vi "run_weather.vi"() -> ()   [LabVIEW 2011]
uses:
  <vilib>/xml/Load XML File.vi
  <vilib>/xml/Close Reference(Node).vi
  Dependencies/global.vi
  <vilib>/xml/NI_XML.lvlib
panel:
  out "SolarRadiation":string
  out "Error File Write":errorcluster
  out "Error Image Convert":errorcluster
  out "+4 Day Hourly Forecast":string[][](array[string])
  out "+3 Day Hourly Forecast":string[][](array[string])
  out "+2 Day Hourly Forecast":string[][](array[string])
  out "+1 Day Hourly Forecast":string[][](array[string])
  in  "File Path":string="C:\\HVAC\\weather.xml"
  out "Error Msg":string
  out "Updating Weather":bool
  out "?":picture
  out "Today Hourly Forecast":string[][](array[string])
  in  "Update Interval (minutes)":dbl=30.0
  out "Now":string[][](array[string])
  out "Observation Time (RFC 822)":string
  out "Elevation":string
  out "Longitude":string
  out "Latitude":string
  out "Country (ISO 3166)":string
  out "Location":string
  in  "City":string="stockholm"
  in  "Country":string="sweden"
  out "URL":string
  out "Key ID":string="3b63fd7c50251341"
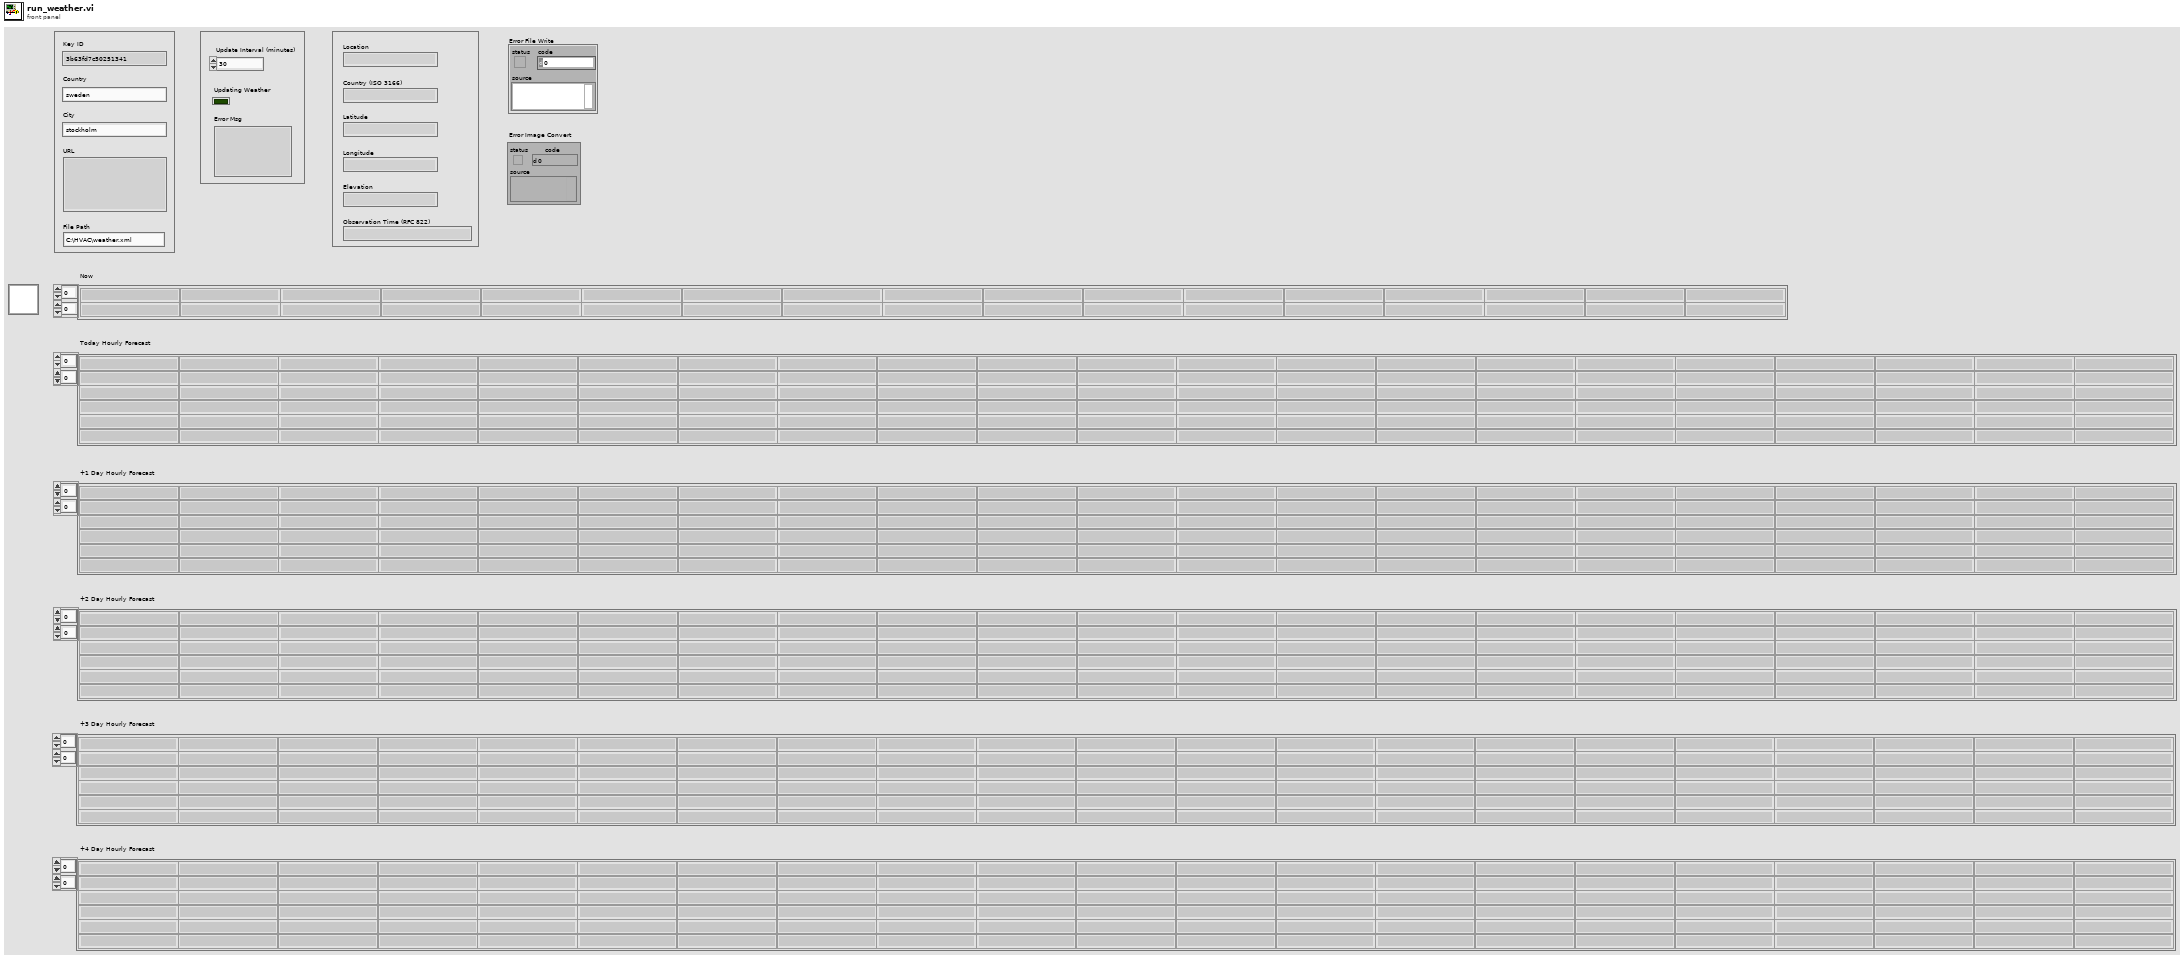
[diagram p1: front panel]
types:
  T1 = cluster{string, string, string, string, string, string, string, string}
  T2 = enum16{"open", "open or create", "create or replace", "create", "open (read only)"}
  T3 = typedef "imagedata.ctl" = cluster{"image type":i32, "image depth":i32, "image":u8[], "mask":u8[], "colors":u32[], "Rectangle":cluster{"left":i16, "top":i16, "right":i16, "bottom":i16}}
  T4 = cluster{string, string, string, string, string, "date/time string":string, string, string}
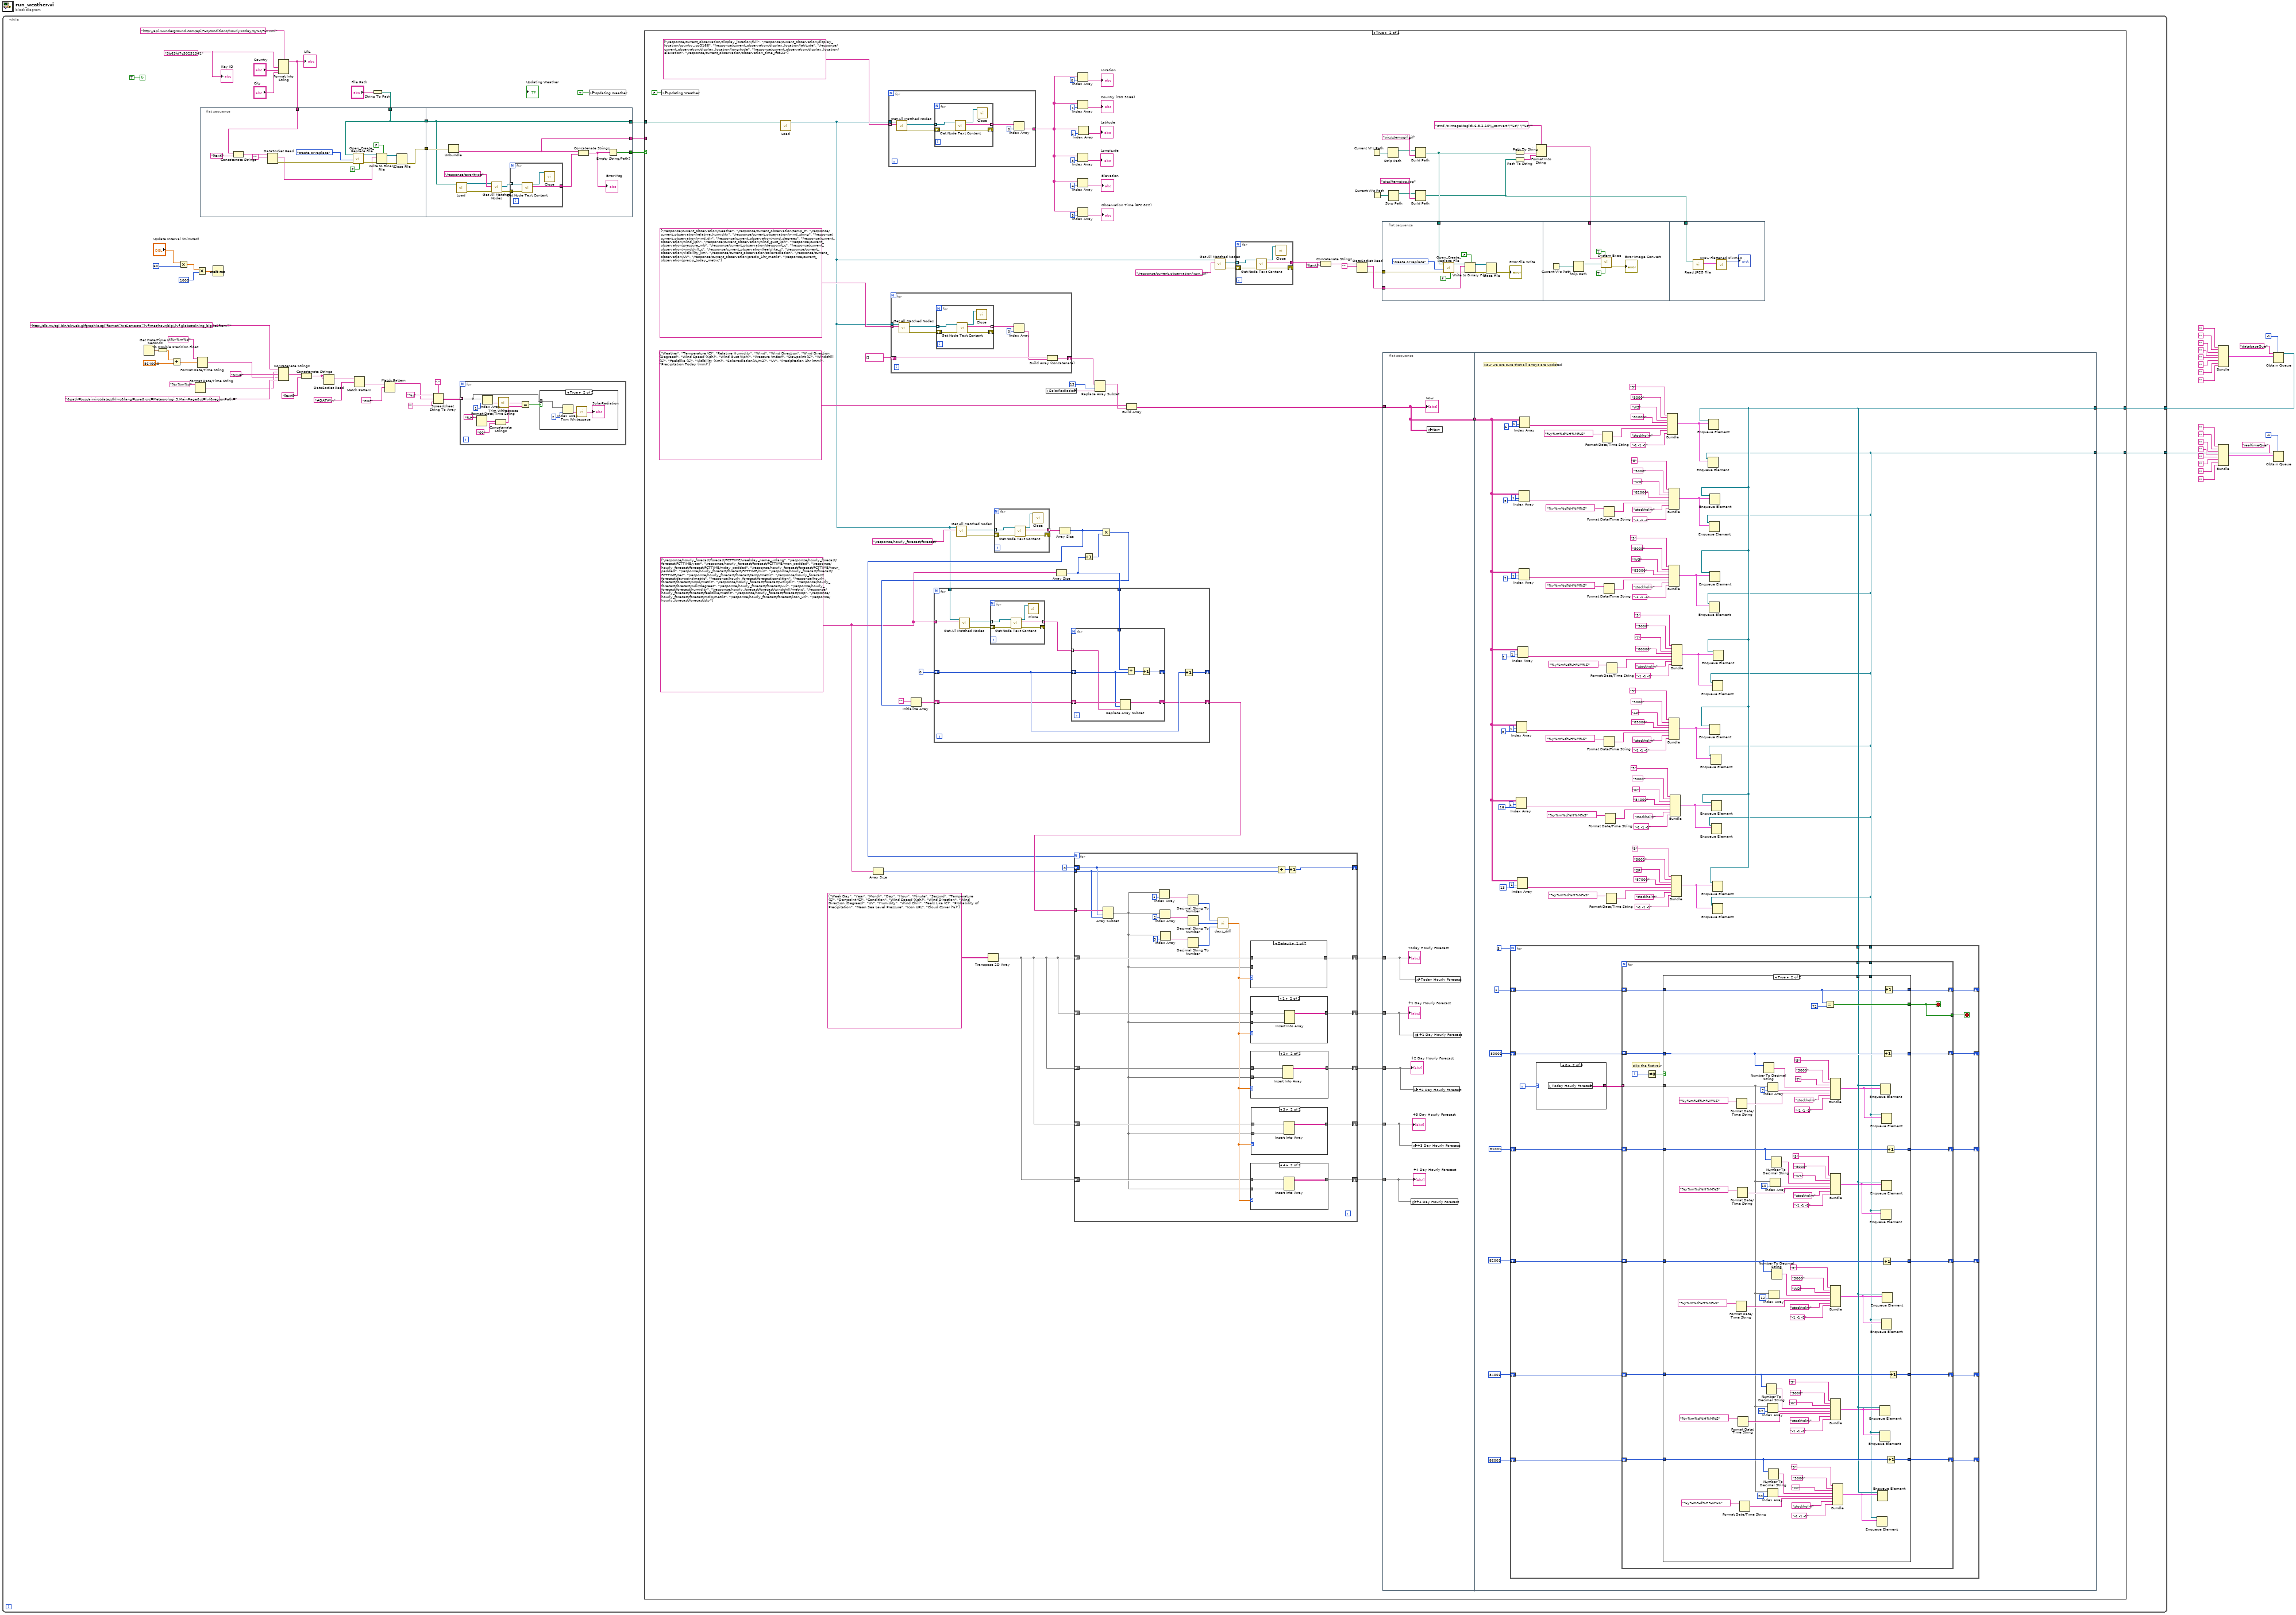
[diagram p0: block diagram]
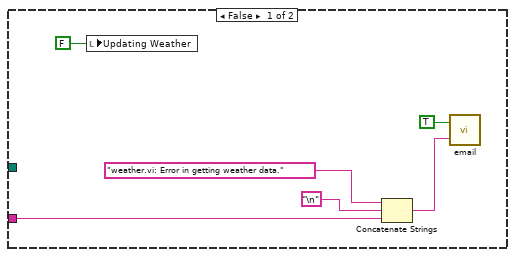
[diagram p3: hidden frame]
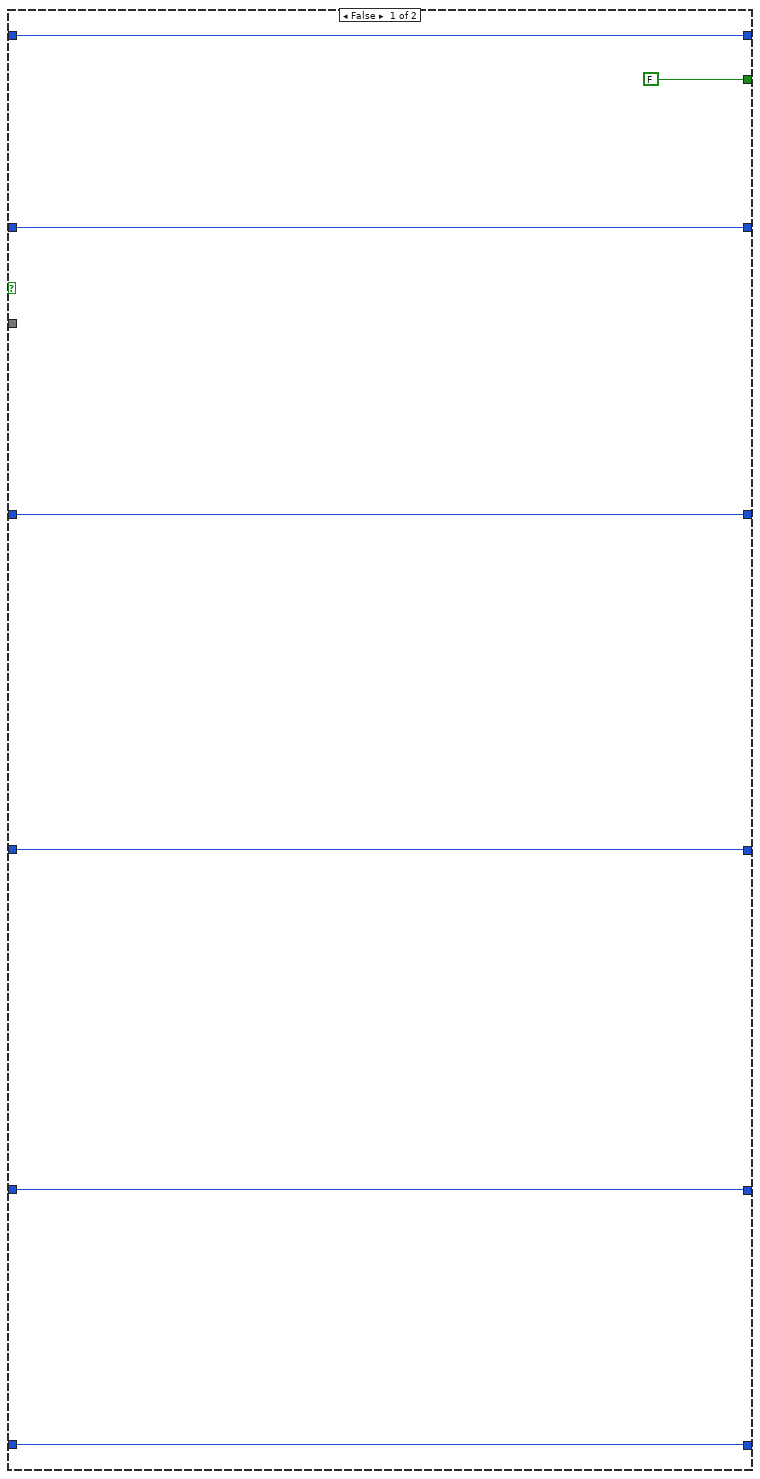
[diagram p4: hidden frame]
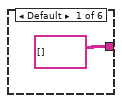
[diagram p5: hidden frame]
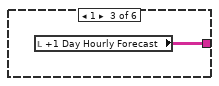
[diagram p6: hidden frame]
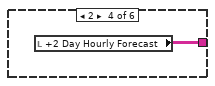
[diagram p7: hidden frame]
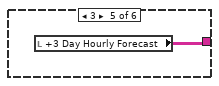
[diagram p8: hidden frame]
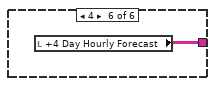
[diagram p9: hidden frame]
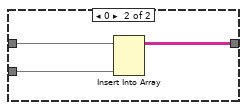
[diagram p14: hidden frame]
diagram:
  n1 = Bundle("", "", "", "", "", "", "", "") -> (w17:T1)  [unwired: 1 in]
  n2 = Bundle("", "", "", "", "", "", "", "") -> (w6:T1)  [unwired: 1 in]
  n3 = Obtain Queue(max queue size (-1, unlimited)=-1, name (unnamed)="databaseQue", element data type=w17) -> (queue out=w2:refnum<queue>)  [unwired: 2 in, 2 out]
  n4 = Obtain Queue(max queue size (-1, unlimited)=-1, name (unnamed)="realtimeQue", element data type=w6) -> (queue out=w1:refnum<queue>)  [unwired: 2 in, 2 out]
  n5 = while {
    tunnel: w2 -> [w49]
    tunnel: w1 -> [w48]
    stop <- TRUE continue-if-true
    w67 = "3b63fd7c50251341"
    n6 = Get Date/Time In Seconds() -> (seconds since 1Jan1904=w34:timestamp)
    n7 = To Double Precision Float(number=w34) -> (double precision float=w33:dbl)
    n8 = Add(x=w33, y=86400.0) -> (x+y=w31:dbl)
    n9 = Multiply(x="Update Interval (minutes)", y=60) -> (x*y=w64:dbl)
    n10 = Format Date/Time String(time format string (%c)="%y%m%d") -> (date/time string=w28:string)  [unwired: 2 in]
    n11 = Multiply(x=w64, y=1000) -> (x*y=w62:dbl)
    n12 = Format Date/Time String(time format string (%c)="%y%m%d", seconds (now)=w31) -> (date/time string=w27:string)  [unwired: 1 in]
    n13 = flat-sequence {
      tunnel: w50 -> [w83]
      tunnel: [w83] -> w57
      tunnel: [w82] -> w56
      tunnel: w53 -> [w86]
      tunnel: w57 -> [w99]
      tunnel: w56 -> [w100]
      tunnel: [w99] -> w55
      tunnel: [w98] -> w54
      tunnel: [w97] -> w52
      frame #0 {
        n14 = Concatenate Strings(w86, "[text]" ("string")) -> (w89:string)
        n15 = DataSocket Read(10:"", 11:w89) -> (0:w85:errorcluster, 2:w84:string)  [unwired: 3 in, 5 out]
        n16 = call <vilib>:"Open_Create_Replace File.vi"("advisory dialog? (display:T)"=FALSE, "error in (no error)"=w85, "function (open:0)"=T2."create or replace", "file path"=w83) -> ("error out"=w92:errorcluster, "refnum"=w91:refnum<file>)  [unwired: 3 in, 3 out]
        n17 = Write to Binary File(file (use dialog)=w91, data=w84, error in=w92, 5:FALSE ("prepend array or string size? (T)")) -> (refnum out=w95:refnum<file>, error out=w96:errorcluster)  [unwired: 3 out]
        n18 = Close File(refnum=w95, error in=w96) -> (error out=w82:errorcluster)  [unwired: 1 out]
      }
      frame #1 {
        n19 = Unbundle(w100) -> ("source"=w97:string)  [unwired: 2 out]
        n20 = call-poly <vilib>:"Load.vi"("path to XML document"=w99) -> ("DOM document out"=w105:refnum<k20>, "error out"=w104:errorcluster)  [unwired: 12 in, 1 out]
        n21 = call <vilib>:"Get All Matched Nodes.vi"("error in (no error)"=w104, "XPath expression"="/response/error/type", "node in"=w105) -> ("error out"=w107:errorcluster, "node result array"=w103:refnum<k20>[])  [unwired: 7 out]
        n22 = for {
          tunnel: w107 -> [w111]
          tunnel: [w110] -> w101
          tunnel: w103 -> [w108] mode=indexing
          n23 = call <vilib>:"Get Node Text Content.vi"("error in (no error)"=w111, "node in"=w108) -> ("node text"=w110:string, "node out"=w109:refnum<k20>)  [unwired: 7 in, 1 out]
          n24 = call-poly <vilib>:"Close.vi"("node"=w109) -> ()  [unwired: 8 in, 1 out]
        }
        n25 = Concatenate Strings(w97, w101) -> (w102:string)
        "Error Msg" <- w102
        n26 = Empty String/Path?(string/path=w102) -> (empty?=w98:bool)
      }
    }
    n27 = Wait (ms)(milliseconds to wait=w62) -> ()  [unwired: 1 out]
    n28 = Format Into String(format string="http://api.wunderground.com/api/%s/conditions/hourly10day/q/%s/%s.xml", w67, "Country", "City") -> (resulting string=w53:string)  [unwired: 2 in, 1 out]
    "URL" <- w53
    n29 = Concatenate Strings("http://slb.nu/cgi-bin/airweb.gifgraphic.cgi?format=txt&zmacro=lvf/met/hour/big//lvf-globstralning_big.ic&from=" ("string"), w28, "&to=" ("string"), w27, "&path=/usr/airviro/data/sthlm/&lang=swe&rsrc=Meteorologi.3.MainPage&st=lvf&regionPath=" ("string")) -> (w38:string)
    n30 = Concatenate Strings(w38, "[text]" ("string")) -> (w46:string)
    n31 = DataSocket Read(10:w46, 11:w46) -> (2:w45:string)  [unwired: 3 in, 6 out]
    n32 = Match Pattern(string=w45, regular expression="#DATA\\n") -> (after substring=w37:string)  [unwired: 1 in, 3 out]
    n33 = String To Path(string="File Path") -> (path=w50:path)
    n34 = Match Pattern(string=w37, regular expression="EOF") -> (before substring=w25:string)  [unwired: 1 in, 3 out]
    n35 = Spreadsheet String To Array(delimiter (Tab)=",", format string="%s", spreadsheet string=w25, array type (2D Dbl)="") -> (array=w26:string[][])
    n36 = for {
      tunnel: w26 -> [w71] mode=indexing
      n37 = Format Date/Time String(time format string (%c)="%H") -> (date/time string=w75:string)  [unwired: 2 in]
      n38 = Index Array(array=w71, index=1) -> (element=w70:string)
      n39 = Concatenate Strings(w75, "00" ("string")) -> (w73:string)
      n40 = call <vilib>:"Trim Whitespace.vi"("string"=w70) -> ("trimmed string"=w69:string)  [unwired: 1 in]
      n41 = Equal?(x=w69, y=w73) -> (x = y?=w72:bool)
      n42 = case shown="True" w72 {
        tunnel: w71 -> [_ w81]
        frame False {
        }
        frame True {
          n43 = Index Array(array=w81, index=2) -> (element=w78:string)
          n44 = call <vilib>:"Trim Whitespace.vi"("string"=w78) -> ("trimmed string"=→"SolarRadiation":string)  [unwired: 1 in]
        }
      }
    }
    n45 = local write "Updating Weather"(TRUE ("Backup in Progress")) -> ()
    n46 = case shown="True" w54 {
      tunnel: w55 -> [_ w188]
      tunnel: w52 -> [w113 _]
      tunnel: w49 -> [_ w123]
      tunnel: w48 -> [_ w122]
      frame False {
        n47 = local write "Updating Weather"(FALSE ("Updating Weather")) -> ()
        n48 = Concatenate Strings("weather.vi: Error in getting weather data.", "\n", w113) -> (w112:string)
        n49 = call "email.vi"("Body"=w112, "Enable"=TRUE) -> ()  [unwired: 1 in]
      }
      frame True {
        w141 = string[] ["/response/hourly_forecast/forecast/FCTTIME/weekday_name_unlang", "/response/hourly_forecast/forecast/FCTTIME/year", "/response/hourly_forecast/forecast/FCTTIME/mon_padded", "/response/hourly_forecast/forecast/FCTTIME/mday_padded", "/response/hourly_forecast/forecast/FCTTIME/hour_padded", "/response/hourly_forecast/forecast/FCTTIME/min", "/response/hourly_forecast/forecast/FCTTIME/sec", "/response/hourly_forecast/forecast/temp/metric", "/response/hourly_forecast/forecast/dewpoint/metric", "/response/hourly_forecast/forecast/condition", "/response/hourly_forecast/forecast/wspd/metric", "/response/hourly_forecast/forecast/wdir/dir", "/response/hourly_forecast/forecast/wdir/degrees", "/response/hourly_forecast/forecast/uvi", "/response/hourly_forecast/forecast/humidity", "/response/hourly_forecast/forecast/windchill/metric", "/response/hourly_forecast/forecast/feelslike/metric", "/response/hourly_forecast/forecast/pop", "/response/hourly_forecast/forecast/mslp/metric", "/response/hourly_forecast/forecast/icon_url", "/response/hourly_forecast/forecast/sky"]
        n50 = local write "Updating Weather"(FALSE ("Backup in Progress")) -> ()
        n51 = call-poly <vilib>:"Load.vi"("path to XML document"=w188) -> ("DOM document out"=w125:refnum<k20>)  [unwired: 12 in, 2 out]
        n52 = Array Size(array=w141) -> (size(s)=w140:i32)
        n53 = for {
          tunnel: string[] ["/response/current_observation/display_location/full", "/response/current_observation/display_location/country_iso3166", "/response/current_observation/display_location/latitude", "/response/current_observation/display_location/longitude", "/response/current_observation/display_location/elevation", "/response/current_observation/observation_time_rfc822"] -> [w526] mode=indexing
          tunnel: w125 -> [w525]
          tunnel: [w521] -> w179 mode=indexing
          n54 = call <vilib>:"Get All Matched Nodes.vi"("XPath expression"=w526, "node in"=w525) -> ("error out"=w524:errorcluster, "node result array"=w527:refnum<k20>[])  [unwired: 1 in, 7 out]
          n55 = for {
            tunnel: w527 -> [w532] mode=indexing
            tunnel: [w531] -> w523 mode=indexing
            shift-right: [w529] -> _
            shift-left: w524 -> [w530]
            n56 = call <vilib>:"Get Node Text Content.vi"("error in (no error)"=w530, "node in"=w532) -> ("error out"=w529:errorcluster, "node text"=w531:string, "node out"=w528:refnum<k20>)  [unwired: 7 in]
            n57 = call-poly <vilib>:"Close.vi"("node"=w528) -> ()  [unwired: 8 in, 1 out]
          }
          n58 = Index Array(array=w523, index=0) -> (element=w521:string)
        }
        n59 = for {
          tunnel: string[] ["/response/current_observation/weather", "/response/current_observation/temp_c", "/response/current_observation/relative_humidity", "/response/current_observation/wind_string", "/response/current_observation/wind_dir", "/response/current_observation/wind_degrees", "/response/current_observation/wind_kph", "/response/current_observation/wind_gust_kph", "/response/current_observation/pressure_mb", "/response/current_observation/dewpoint_c", "/response/current_observation/windchill_c", "/response/current_observation/feelslike_c", "/response/current_observation/visibility_km", "/response/current_observation/solarradiation", "/response/current_observation/UV", "/response/current_observation/precip_1hr_metric", "/response/current_observation/precip_today_metric"] -> [w514] mode=indexing
          shift-right: [w510] -> w121
          shift-left: string[] [] -> [w509]
          tunnel: w125 -> [w507]
          n60 = call <vilib>:"Get All Matched Nodes.vi"("XPath expression"=w514, "node in"=w507) -> ("error out"=w513:errorcluster, "node result array"=w515:refnum<k20>[])  [unwired: 1 in, 7 out]
          n61 = for {
            tunnel: w515 -> [w520] mode=indexing
            tunnel: [w519] -> w512 mode=indexing
            shift-right: [w517] -> _
            shift-left: w513 -> [w518]
            n62 = call <vilib>:"Get Node Text Content.vi"("error in (no error)"=w518, "node in"=w520) -> ("error out"=w517:errorcluster, "node text"=w519:string, "node out"=w516:refnum<k20>)  [unwired: 7 in]
            n63 = call-poly <vilib>:"Close.vi"("node"=w516) -> ()  [unwired: 8 in, 1 out]
          }
          n64 = Index Array(array=w512, index=0) -> (element=w508:string)
          n65 = Build Array (concatenate)(w509, w508) -> (w510:string[])
        }
        n66 = call <vilib>:"Get All Matched Nodes.vi"("XPath expression"="/response/hourly_forecast/forecast", "node in"=w125) -> ("error out"=w168:errorcluster, "node result array"=w167:refnum<k20>[])  [unwired: 1 in, 7 out]
        n67 = Transpose 2D Array(2D array=string[][] [["Week Day"], ["Year"], ["Month"], ["Day"], ["Hour"], ["Minute"], ["Second"], ["Temperature (C)"], ["Dewpoint (C)"], ["Condition"], ["Wind Speed (Kph)"], ["Wind Direction"], ["Wind Direction (Degrees)"], ["UV"], ["Humidity"], ["Wind Chill"], ["Feels Like (C)"], ["Probability of Precipitation"], ["Mean Sea Level Pressure"], ["Icon URL"], ["Cloud Cover (%)"]]) -> (transposed array=w132:string[][])
        n68 = for {
          tunnel: w167 -> [w484] mode=indexing
          tunnel: [w483] -> w165 mode=indexing
          shift-right: [w481] -> _
          shift-left: w168 -> [w482]
          n69 = call <vilib>:"Get Node Text Content.vi"("error in (no error)"=w482, "node in"=w484) -> ("error out"=w481:errorcluster, "node text"=w483:string, "node out"=w480:refnum<k20>)  [unwired: 7 in]
          n70 = call-poly <vilib>:"Close.vi"("node"=w480) -> ()  [unwired: 8 in, 1 out]
        }
        n71 = local read "SolarRadiation"() -> (w120:string)
        n72 = Array Size(array=w141) -> (size(s)=w164:i32)
        n73 = Array Size(array=w165) -> (size(s)=w139:i32)
        n74 = Index Array(array=w179, index=0) -> (element=→"Location":string)
        n75 = Index Array(array=w179, index=1) -> (element=→"Country (ISO 3166)":string)
        n76 = Index Array(array=w179, index=3) -> (element=→"Longitude":string)
        n77 = Index Array(array=w179, index=4) -> (element=→"Elevation":string)
        n78 = Index Array(array=w179, index=5) -> (element=→"Observation Time (RFC 822)":string)
        n79 = Index Array(array=w179, index=2) -> (element=→"Latitude":string)
        n80 = Increment(x=w164) -> (x+1=w163:i32)
        n81 = Replace Array Subset(array=w121, new element=w120, index=13) -> (w118:string[])
        n82 = Multiply(x=w139, y=w163) -> (x*y=w162:i32)
        n83 = Initialize Array("", w162) -> (w169:string[])
        n84 = for {
          tunnel: w141 -> [w493] mode=indexing
          tunnel: w125 -> [w491]
          shift-right: [w485] -> w143
          shift-left: w169 -> [w486]
          tunnel: w164 -> [w489]
          shift-right: [w488] -> _
          shift-left: 0 -> [w487]
          n85 = call <vilib>:"Get All Matched Nodes.vi"("XPath expression"=w493, "node in"=w491) -> ("error out"=w492:errorcluster, "node result array"=w494:refnum<k20>[])  [unwired: 1 in, 7 out]
          n86 = for {
            tunnel: w494 -> [w506] mode=indexing
            tunnel: [w505] -> w490 mode=indexing
            shift-right: [w503] -> _
            shift-left: w492 -> [w504]
            n87 = call <vilib>:"Get Node Text Content.vi"("error in (no error)"=w504, "node in"=w506) -> ("error out"=w503:errorcluster, "node text"=w505:string, "node out"=w502:refnum<k20>)  [unwired: 7 in]
            n88 = call-poly <vilib>:"Close.vi"("node"=w502) -> ()  [unwired: 8 in, 1 out]
          }
          n89 = for {
            tunnel: w490 -> [w495] mode=indexing
            shift-right: [w499] -> _
            shift-left: w487 -> [w497]
            tunnel: w489 -> [w501]
            shift-right: [w496] -> w485
            shift-left: w486 -> [w498]
            n90 = Replace Array Subset(array=w498, new element=w495, index=w497) -> (w496:string[])
            n91 = Add(x=w501, y=w497) -> (x+y=w500:i32)
            n92 = Increment(x=w500) -> (x+1=w499:i32)
          }
          n93 = Increment(x=w487) -> (x+1=w488:i32)
        }
        n94 = for {
          N: w139 -> [_]
          tunnel: w143 -> [w434]
          shift-right: [w423] -> w137
          shift-left: w132 -> [w424]
          shift-right: [w421] -> w138
          shift-left: w132 -> [w422]
          shift-right: [w419] -> _
          shift-left: u64 0 -> [w418]
          tunnel: w140 -> [w417]
          shift-right: [w412] -> w136
          shift-left: w132 -> [w415]
          shift-right: [w411] -> w135
          shift-left: w132 -> [w414]
          shift-right: [w410] -> w134
          shift-left: w132 -> [w413]
          n95 = Array Subset(array=w434, index=w418, length=w417) -> (w409:string[])
          n96 = Index Array(array=w409, index=1 ("index (row)")) -> (element=w430:string)
          n97 = Index Array(array=w409, index=2 ("index (row)")) -> (element=w429:string)
          n98 = Index Array(array=w409, index=3 ("index (row)")) -> (element=w428:string)
          n99 = Decimal String To Number(string=w430) -> (number=w427:i32)  [unwired: 2 in, 1 out]
          n100 = Decimal String To Number(string=w429) -> (number=w426:i32)  [unwired: 2 in, 1 out]
          n101 = Decimal String To Number(string=w428) -> (number=w425:i32)  [unwired: 2 in, 1 out]
          n102 = call "days_diff.vi"("day"=w425, "month"=w426, "year"=w427) -> ("Days Diff"=w416:dbl)  [unwired: 2 out]
          n103 = case shown="Default" w416 {
            tunnel: w424 -> [w451 w454]
            tunnel: w409 -> [_ w453]
            tunnel: [w451 w452] -> w423
            frame Default {
            }
            frame 0 {
              n104 = Insert Into Array(array=w454, new element=w453) -> (w452:string[][])  [unwired: 2 in]
            }
          }
          n105 = case shown="1" w416 {
            tunnel: w422 -> [w447 w450]
            tunnel: w409 -> [_ w449]
            tunnel: [w447 w448] -> w421
            frame Default {
            }
            frame 1 {
              n106 = Insert Into Array(array=w450, new element=w449) -> (w448:string[][])  [unwired: 2 in]
            }
          }
          n107 = case shown="4" w416 {
            tunnel: w413 -> [w435 w438]
            tunnel: w409 -> [_ w437]
            tunnel: [w435 w436] -> w410
            frame Default {
            }
            frame 4 {
              n108 = Insert Into Array(array=w438, new element=w437) -> (w436:string[][])  [unwired: 2 in]
            }
          }
          n109 = case shown="2" w416 {
            tunnel: w415 -> [w443 w446]
            tunnel: w409 -> [_ w445]
            tunnel: [w443 w444] -> w412
            frame Default {
            }
            frame 2 {
              n110 = Insert Into Array(array=w446, new element=w445) -> (w444:string[][])  [unwired: 2 in]
            }
          }
          n111 = case shown="3" w416 {
            tunnel: w414 -> [w439 w442]
            tunnel: w409 -> [_ w441]
            tunnel: [w439 w440] -> w411
            frame Default {
            }
            frame 3 {
              n112 = Insert Into Array(array=w442, new element=w441) -> (w440:string[][])  [unwired: 2 in]
            }
          }
          n113 = Add(x=w418, y=w417) -> (x+y=w420:u64)
          n114 = Increment(x=w420) -> (x+1=w419:u64)
        }
        n115 = Build Array(string[] ["Weather", "Temperature (C)", "Relative Humidity", "Wind", "Wind Direction", "Wind Direction (Degrees)", "Wind Speed (Kph)", "Wind Gust (Kph)", "Pressure (mBar)", "Dewpoint (C)", "Windchill (C)", "Feelslike (C)", "Visibility (Km)", "Solarradiation(W/m2)", "UV", "Precipitation 1hr (mm)", "Precipitation Today (mm)"], w118) -> (w126:string[][])
        n116 = call <vilib>:"Get All Matched Nodes.vi"("XPath expression"="/response/current_observation/icon_url", "node in"=w125) -> ("error out"=w161:errorcluster, "node result array"=w160:refnum<k20>[])  [unwired: 1 in, 7 out]
        n117 = for {
          tunnel: w160 -> [w479] mode=indexing
          tunnel: [w478] -> w155
          shift-right: [w476] -> _
          shift-left: w161 -> [w477]
          n118 = call <vilib>:"Get Node Text Content.vi"("error in (no error)"=w477, "node in"=w479) -> ("error out"=w476:errorcluster, "node text"=w478:string, "node out"=w475:refnum<k20>)  [unwired: 7 in]
          n119 = call-poly <vilib>:"Close.vi"("node"=w475) -> ()  [unwired: 8 in, 1 out]
        }
        n120 = Concatenate Strings(w155, "[text]" ("string")) -> (w153:string)
        n121 = DataSocket Read(10:"", 11:w153) -> (0:w156:errorcluster, 2:w158:string)  [unwired: 3 in, 5 out]
        n122 = Current VI's Path() -> (path=w131:path)
        n123 = Current VI's Path() -> (path=w129:path)
        n124 = flat-sequence {
          tunnel: w158 -> [w463]
          tunnel: w156 -> [w460]
          tunnel: w150 -> [w456]
          tunnel: w145 -> [w467]
          tunnel: w147 -> [w472]
          frame #0 {
            n125 = call <vilib>:"Open_Create_Replace File.vi"("advisory dialog? (display:T)"=FALSE, "error in (no error)"=w460, "function (open:0)"=T2."create or replace", "file path"=w456) -> ("error out"=w462:errorcluster, "refnum"=w464:refnum<file>)  [unwired: 3 in, 3 out]
            n126 = Write to Binary File(file (use dialog)=w464, data=w463, error in=w462, 5:FALSE ("prepend array or string size? (T)")) -> (refnum out=w458:refnum<file>, error out=w457:errorcluster)  [unwired: 3 out]
            n127 = Close File(refnum=w458, error in=w457) -> (error out=→"Error File Write":errorcluster)  [unwired: 1 out]
          }
          frame #1 {
            n128 = Current VI's Path() -> (path=w468:path)
            n129 = Strip Path(path=w468) -> (stripped path=w471:path)  [unwired: 1 out]
            n130 = call <vilib>:"System Exec.vi"("run minimized? (F)"=TRUE, "wait until completion? (T)"=TRUE, "working directory"=w471, "command line"=w467) -> ("error out"=→"Error Image Convert":errorcluster)  [unwired: 4 in, 3 out]
          }
          frame #2 {
            n131 = call <vilib>:"Read JPEG File.vi"("path to JPEG file"=w472) -> ("image data"=w473:T3)  [unwired: 8 in, 2 out]
            n132 = call <vilib>:"Draw Flattened Pixmap.vi"("image data"=w473) -> ("new picture"=→"?":picture)  [unwired: 3 in, 5 out]
          }
        }
        n133 = flat-sequence {
          tunnel: w138 -> [w194]
          tunnel: w137 -> [w193]
          tunnel: w136 -> [w192]
          tunnel: w135 -> [w191]
          tunnel: w134 -> [w190]
          tunnel: w126 -> [w189]
          tunnel: [w189] -> w124
          tunnel: w124 -> [w197]
          tunnel: w123 -> [w196]
          tunnel: w122 -> [w195]
          frame #0 {
            n134 = global write "global.vi" "+4 Day Hourly Forecast"(w190) -> ()
            n135 = global write "global.vi" "+3 Day Hourly Forecast"(w191) -> ()
            n136 = global write "global.vi" "+2 Day Hourly Forecast"(w192) -> ()
            n137 = global write "global.vi" "+1 Day Hourly Forecast"(w194) -> ()
            n138 = global write "global.vi" "Today Hourly Forecast"(w193) -> ()
            n139 = global write "global.vi" "Now"(w189) -> ()
            "Now" <- w189
            "Today Hourly Forecast" <- w193
            "+1 Day Hourly Forecast" <- w194
            "+2 Day Hourly Forecast" <- w192
            "+3 Day Hourly Forecast" <- w191
            "+4 Day Hourly Forecast" <- w190
          }
          frame #1 {
            # "Now we are sure that all arrays are updated"
            n140 = for {
              N: 5 -> [_]
              shift-right: [w301] -> _
              shift-left: 80001 -> [w302]
              tunnel: w196 -> [w304]
              shift-right: [w299] -> _
              shift-left: 81001 -> [w300]
              shift-right: [w297] -> _
              shift-left: 82001 -> [w298]
              shift-right: [w295] -> _
              shift-left: 84001 -> [w296]
              shift-right: [w293] -> _
              shift-left: 1 -> [w294]
              shift-right: [w291] -> _
              shift-left: 86001 -> [w290]
              tunnel: w195 -> [w289]
              i -> [w305]
              stop <- w292 stop-if-true
              n141 = case shown="0" w305 {
                tunnel: [string[][] [] ("Today Hourly Forecast") w404 w405 w406 w407 w408] -> w303
                frame Default {
                }
                frame 0 {
                  n142 = local read "Today Hourly Forecast"() -> (w404:string[][])
                }
                frame 1 {
                  n143 = local read "+1 Day Hourly Forecast"() -> (w405:string[][])
                }
                frame 2 {
                  n144 = local read "+2 Day Hourly Forecast"() -> (w406:string[][])
                }
                frame 3 {
                  n145 = local read "+3 Day Hourly Forecast"() -> (w407:string[][])
                }
                frame 4 {
                  n146 = local read "+4 Day Hourly Forecast"() -> (w408:string[][])
                }
              }
              n147 = for {
                tunnel: w304 -> [w321]
                tunnel: w303 -> [w320] mode=indexing
                shift-right: [w318] -> w301
                shift-left: w302 -> [w319]
                shift-right: [w316] -> w299
                shift-left: w300 -> [w317]
                shift-right: [w315] -> w297
                shift-left: w298 -> [w314]
                shift-right: [w313] -> w295
                shift-left: w296 -> [w312]
                shift-right: [w310] -> w293
                shift-left: w294 -> [w311]
                tunnel: [w309] -> w292
                shift-right: [w307] -> w291
                shift-left: w290 -> [w308]
                tunnel: w289 -> [w306]
                i -> [w323]
                stop <- w309 stop-if-true
                # "skip the first row"
                n148 = Not Equal To 0?(x=w323) -> (x != 0?=w322:bool)
                n149 = case shown="True" w322 {
                  tunnel: [w330 w401] -> w318
                  tunnel: w319 -> [w330 w397]
                  tunnel: w321 -> [_ w338]
                  tunnel: w320 -> [_ w337]
                  tunnel: w317 -> [w329 w392]
                  tunnel: [w329 w391] -> w316
                  tunnel: [w328 w386] -> w315
                  tunnel: w314 -> [w328 w385]
                  tunnel: [w327 w380] -> w313
                  tunnel: w312 -> [w327 w379]
                  tunnel: w311 -> [w326 w376]
                  tunnel: [w326 w377] -> w310
                  tunnel: [FALSE w375] -> w309
                  tunnel: w308 -> [w324 w340]
                  tunnel: [w324 w339] -> w307
                  tunnel: w306 -> [_ w331]
                  frame False {
                  }
                  frame True {
                    n150 = Format Date/Time String(time format string (%c)="%y%m%d%H%M%S") -> (date/time string=w368:string)  [unwired: 2 in]
                    n151 = Format Date/Time String(time format string (%c)="%y%m%d%H%M%S") -> (date/time string=w373:string)  [unwired: 2 in]
                    n152 = Format Date/Time String(time format string (%c)="%y%m%d%H%M%S") -> (date/time string=w369:string)  [unwired: 2 in]
                    n153 = Format Date/Time String(time format string (%c)="%y%m%d%H%M%S") -> (date/time string=w367:string)  [unwired: 2 in]
                    n154 = Format Date/Time String(time format string (%c)="%y%m%d%H%M%S") -> (date/time string=w345:string)  [unwired: 2 in]
                    n155 = Number To Decimal String(number=w397) -> (decimal integer string=w363:string)  [unwired: 1 in]
                    n156 = Number To Decimal String(number=w379) -> (decimal integer string=w351:string)  [unwired: 1 in]
                    n157 = Index Array(array=w337, index=17) -> (element=w384:string)
                    n158 = Index Array(array=w337, index=20) -> (element=w350:string)
                    n159 = Index Array(array=w337, index=7) -> (element=w398:string)
                    n160 = Number To Decimal String(number=w340) -> (decimal integer string=w341:string)  [unwired: 1 in]
                    n161 = Index Array(array=w337, index=12) -> (element=w387:string)
                    n162 = Index Array(array=w337, index=10) -> (element=w396:string)
                    n163 = Number To Decimal String(number=w392) -> (decimal integer string=w359:string)  [unwired: 1 in]
                    n164 = Number To Decimal String(number=w385) -> (decimal integer string=w355:string)  [unwired: 1 in]
                    n165 = Equal?(x=w376, y=72) -> (x = y?=w375:bool)
                    n166 = Bundle("5", "5000", "T", w363, w398, "date/time string"=w373, "stockholm", "-1 -1 -1") -> (w336:T4)  [unwired: 1 in]
                    n167 = Bundle("5", "5000", "WS", w359, w396, "date/time string"=w369, "stockholm", "-1 -1 -1") -> (w335:T4)  [unwired: 1 in]
                    n168 = Bundle("5", "5000", "WD", w355, w387, "date/time string"=w368, "stockholm", "-1 -1 -1") -> (w334:T4)  [unwired: 1 in]
                    n169 = Bundle("5", "5000", "Pr", w351, w384, "date/time string"=w367, "stockholm", "-1 -1 -1") -> (w333:T4)  [unwired: 1 in]
                    n170 = Bundle("5", "5000", "CC", w341, w350, "date/time string"=w345, "stockholm", "-1 -1 -1") -> (w332:T4)  [unwired: 1 in]
                    n171 = Enqueue Element(queue=w331, element=w332) -> ()  [unwired: 2 in, 3 out]
                    n172 = Enqueue Element(queue=w338, element=w332) -> ()  [unwired: 2 in, 3 out]
                    n173 = Enqueue Element(queue=w331, element=w333) -> ()  [unwired: 2 in, 3 out]
                    n174 = Enqueue Element(queue=w338, element=w333) -> ()  [unwired: 2 in, 3 out]
                    n175 = Enqueue Element(queue=w338, element=w336) -> ()  [unwired: 2 in, 3 out]
                    n176 = Enqueue Element(queue=w331, element=w335) -> ()  [unwired: 2 in, 3 out]
                    n177 = Enqueue Element(queue=w331, element=w336) -> ()  [unwired: 2 in, 3 out]
                    n178 = Enqueue Element(queue=w338, element=w335) -> ()  [unwired: 2 in, 3 out]
                    n179 = Enqueue Element(queue=w331, element=w334) -> ()  [unwired: 2 in, 3 out]
                    n180 = Increment(x=w385) -> (x+1=w386:i32)
                    n181 = Enqueue Element(queue=w338, element=w334) -> ()  [unwired: 2 in, 3 out]
                    n182 = Increment(x=w397) -> (x+1=w401:i32)
                    n183 = Increment(x=w376) -> (x+1=w377:i32)
                    n184 = Increment(x=w392) -> (x+1=w391:i32)
                    n185 = Increment(x=w340) -> (x+1=w339:i32)
                    n186 = Increment(x=w379) -> (x+1=w380:i32)
                  }
                }
              }
            }
            n187 = Index Array(array=w197, index (row)=1 ("index"), index (col)=16 ("disabled index (col)")) -> (element=w251:string)
            n188 = Index Array(array=w197, index (row)=1 ("index"), index (col)=8 ("disabled index (col)")) -> (element=w250:string)
            n189 = Index Array(array=w197, index (row)=1 ("index"), index (col)=13 ("disabled index (col)")) -> (element=w202:string)
            n190 = Index Array(array=w197, index (row)=1 ("index"), index (col)=1 ("disabled index (col)")) -> (element=w242:string)
            n191 = Index Array(array=w197, index (row)=1 ("index"), index (col)=5 ("disabled index (col)")) -> (element=w258:string)
            n192 = Index Array(array=w197, index (row)=1 ("index"), index (col)=7 ("disabled index (col)")) -> (element=w249:string)
            n193 = Index Array(array=w197, index (row)=1 ("index"), index (col)=6 ("disabled index (col)")) -> (element=w281:string)
            n194 = Format Date/Time String(time format string (%c)="%y%m%d%H%M%S") -> (date/time string=w287:string)  [unwired: 2 in]
            n195 = Format Date/Time String(time format string (%c)="%y%m%d%H%M%S") -> (date/time string=w277:string)  [unwired: 2 in]
            n196 = Format Date/Time String(time format string (%c)="%y%m%d%H%M%S") -> (date/time string=w274:string)  [unwired: 2 in]
            n197 = Format Date/Time String(time format string (%c)="%y%m%d%H%M%S") -> (date/time string=w267:string)  [unwired: 2 in]
            n198 = Format Date/Time String(time format string (%c)="%y%m%d%H%M%S") -> (date/time string=w264:string)  [unwired: 2 in]
            n199 = Format Date/Time String(time format string (%c)="%y%m%d%H%M%S") -> (date/time string=w208:string)  [unwired: 2 in]
            n200 = Format Date/Time String(time format string (%c)="%y%m%d%H%M%S") -> (date/time string=w237:string)  [unwired: 2 in]
            n201 = Bundle("5", "5000", "WS", "81000", w281, "date/time string"=w287, "stockholm", "-1 -1 -1") -> (w215:T4)  [unwired: 1 in]
            n202 = Bundle("5", "5000", "WD", "82000", w258, "date/time string"=w277, "stockholm", "-1 -1 -1") -> (w214:T4)  [unwired: 1 in]
            n203 = Bundle("5", "5000", "WG", "83000", w249, "date/time string"=w274, "stockholm", "-1 -1 -1") -> (w213:T4)  [unwired: 1 in]
            n204 = Bundle("5", "5000", "AP", "85000", w250, "date/time string"=w267, "stockholm", "-1 -1 -1") -> (w211:T4)  [unwired: 1 in]
            n205 = Bundle("5", "5000", "Pr", "84000", w251, "date/time string"=w264, "stockholm", "-1 -1 -1") -> (w210:T4)  [unwired: 1 in]
            n206 = Bundle("5", "5001", "SR", "87000", w202, "date/time string"=w208, "stockholm", "-1 -1 -1") -> (w198:T4)  [unwired: 1 in]
            n207 = Bundle("5", "5000", "T", "80000", w242, "date/time string"=w237, "stockholm", "-1 -1 -1") -> (w212:T4)  [unwired: 1 in]
            n208 = Enqueue Element(queue=w195, element=w215) -> ()  [unwired: 2 in, 3 out]
            n209 = Enqueue Element(queue=w196, element=w215) -> ()  [unwired: 2 in, 3 out]
            n210 = Enqueue Element(queue=w195, element=w214) -> ()  [unwired: 2 in, 3 out]
            n211 = Enqueue Element(queue=w195, element=w213) -> ()  [unwired: 2 in, 3 out]
            n212 = Enqueue Element(queue=w196, element=w214) -> ()  [unwired: 2 in, 3 out]
            n213 = Enqueue Element(queue=w196, element=w213) -> ()  [unwired: 2 in, 3 out]
            n214 = Enqueue Element(queue=w196, element=w211) -> ()  [unwired: 2 in, 3 out]
            n215 = Enqueue Element(queue=w195, element=w211) -> ()  [unwired: 2 in, 3 out]
            n216 = Enqueue Element(queue=w196, element=w210) -> ()  [unwired: 2 in, 3 out]
            n217 = Enqueue Element(queue=w195, element=w210) -> ()  [unwired: 2 in, 3 out]
            n218 = Enqueue Element(queue=w195, element=w212) -> ()  [unwired: 2 in, 3 out]
            n219 = Enqueue Element(queue=w196, element=w198) -> ()  [unwired: 2 in, 3 out]
            n220 = Enqueue Element(queue=w195, element=w198) -> ()  [unwired: 2 in, 3 out]
            n221 = Enqueue Element(queue=w196, element=w212) -> ()  [unwired: 2 in, 3 out]
          }
        }
        n222 = Strip Path(path=w131) -> (stripped path=w130:path)  [unwired: 1 out]
        n223 = Strip Path(path=w129) -> (stripped path=w128:path)  [unwired: 1 out]
        n224 = Build Path(base path=w130, name or relative path="pics\\tempgif.gif") -> (appended path=w150:path)
        n225 = Build Path(base path=w128, name or relative path="pics\\tempjpg.jpg") -> (appended path=w147:path)
        n226 = Path To String(path=w150) -> (string=w149:string)
        n227 = Path To String(path=w147) -> (string=w148:string)
        n228 = Format Into String(format string="cmd /c ImageMagick-6.8.2-10\\\\convert \"%s\" \"%s\"", w149, w148) -> (resulting string=w145:string)  [unwired: 2 in, 1 out]
      }
    }
    "Key ID" <- w67
  }
